vi "test.vi"() -> ()   [LabVIEW 2016]
uses:
  Source/JSON Value/New JSON Value/New JSON (String[]).vi
  Source/JSON Value/Array/Append Array Element.vi
  Source/JSON Value/New JSON Value/New JSON ({String[]}).vi
  Source/JSON Value/New JSON Value/New JSON ({Value}).vi
  Source/JSON Value/Object/Insert Value/Insert Value (Value).vi
  Source/JSON Value/New JSON Value/New JSON ([]).vi
  Source/JSON Value/JSON Value.lvclass
panel:
  out "String 2":string
  out "unsigned byte array":u8[](array[numeric])
  out "String":string
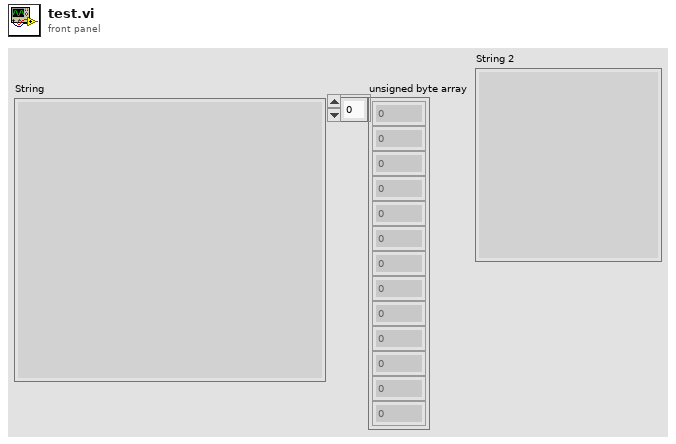
[diagram p1: front panel]
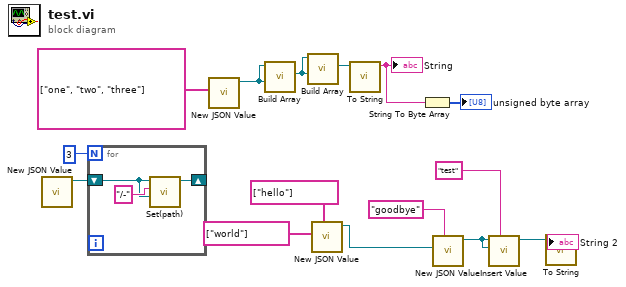
[diagram p0: block diagram]
diagram:
  n1 = call-poly "New JSON Value.vi"() -> ("JSON Value out"=w14:refnum<class "JSON Value.lvclass">)  [unwired: 10 in, 1 out]
  n2 = for {
    N: 3 -> [_]
    shift-right: [w18] -> _
    shift-left: w14 -> [w17]
    n3 = call "Set(path).vi"("value to set"=w17, "Path"="/-", "JSON Value in"=w17) -> ("JSON Value out"=w18:refnum<class "JSON Value.lvclass">)  [unwired: 7 in, 1 out]
  }
  n4 = call-poly "New JSON Value.vi"("String Array"=string[] ["one", "two", "three"]) -> ("JSON Value out"=w13:refnum<class "JSON Value.lvclass">)  [unwired: 9 in, 1 out]
  n5 = call-poly "Build Array.vi"(9:"JSON Value in"=w13, 11:"JSON Value in"=w13) -> ("JSON Value out"=w11:refnum<class "JSON Value.lvclass">)  [unwired: 8 in, 1 out]
  n6 = call-poly "Build Array.vi"(9:"JSON Value in"=w11, 11:"JSON Value in"=w11) -> ("JSON Value out"=w12:refnum<class "JSON Value.lvclass">)  [unwired: 8 in, 1 out]
  n7 = call-poly "New JSON Value.vi"("keys"=string[] ["hello"], "values"=string[] ["world"]) -> ("JSON Value out"=w6:refnum<class "JSON Value.lvclass">)  [unwired: 8 in, 1 out]
  n8 = call "To String.vi"("JSON Value in"=w12) -> ("String"=w10:string)  [unwired: 9 in, 1 out]
  "String" <- w10
  n9 = String To Byte Array(string=w10) -> (unsigned byte array=→"unsigned byte array":u8[])
  n10 = call-poly "New JSON Value.vi"("key"="goodbye", "JSON Value in"=w6) -> ("JSON Value out"=w2:refnum<class "JSON Value.lvclass">)  [unwired: 8 in, 1 out]
  n11 = call-poly "Insert Value.vi"("key"="test", 10:"JSON Value in"=w2, 11:"JSON Value in"=w2) -> ("JSON Value out"=w3:refnum<class "JSON Value.lvclass">)  [unwired: 6 in, 2 out]
  n12 = call "To String.vi"("JSON Value in"=w3) -> ("String"=→"String 2":string)  [unwired: 9 in, 1 out]
